vi "Copy_Template.vi"(1 "报告保存路径":path, 2 "模板路径":path) -> (0 "报告保存路径字符串":string)   [LabVIEW 2015]
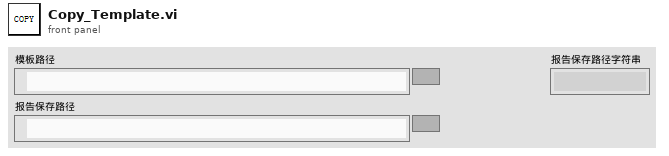
[diagram p1: front panel]
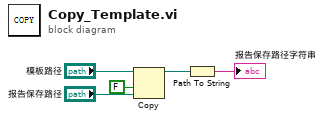
[diagram p0: block diagram]
diagram:
  n1 = Copy(9:FALSE ("overwrite (F)"), 10:"报告保存路径", 11:"模板路径") -> (3:w2:path)  [unwired: 2 in, 2 out]
  n2 = Path To String(path=w2) -> (string=→"报告保存路径字符串":string)
